vi "ExSubNframeCol_new_recovery_no chart.vi"(8 "error in (no error)":errorcluster, 9 "image handles":u32[](array[numeric]), 10 "Number of Images":u32=1 min=1 step=1, 11 "Handle Cluster 2":T1) -> (0 "error out":errorcluster, 1 "data handles":u32[](array[numeric]), 3 "Handle Cluster":T1, 4 "x > y?":bool, 5 "Frame Rate":dbl=1001.0010010010011, 6 "image #":i32)   [LabVIEW 2015]
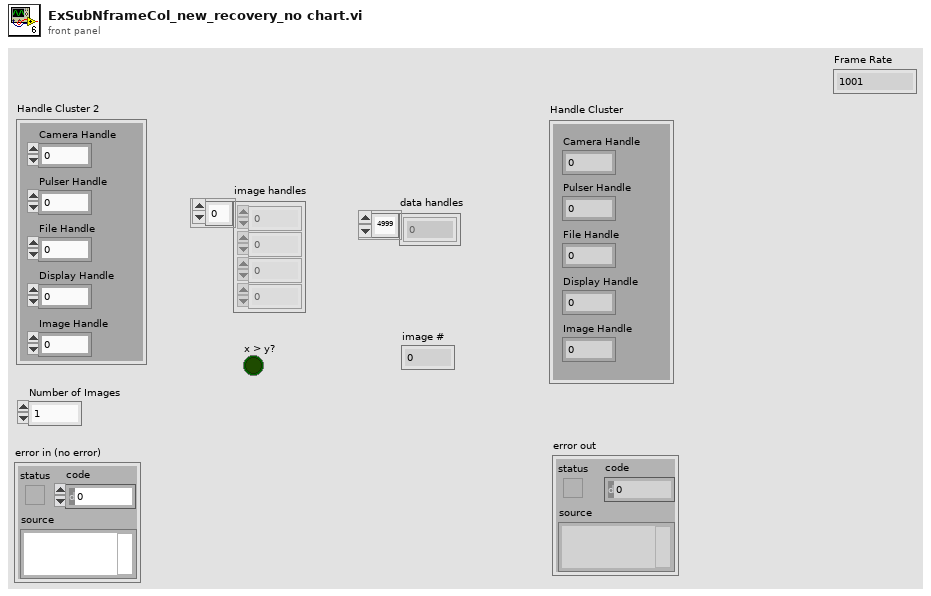
[diagram p1: front panel]
types:
  T1 = cluster{"Camera Handle":u32, "Pulser Handle":u32, "File Handle":u32, "Display Handle":u32, "Image Handle":u32}
  T2 = cluster{"Camera Handle":u32, "Pulser Handle":u32, "File Handle":u32, "Display Handle":u32, "Image/Data Handle":u32}
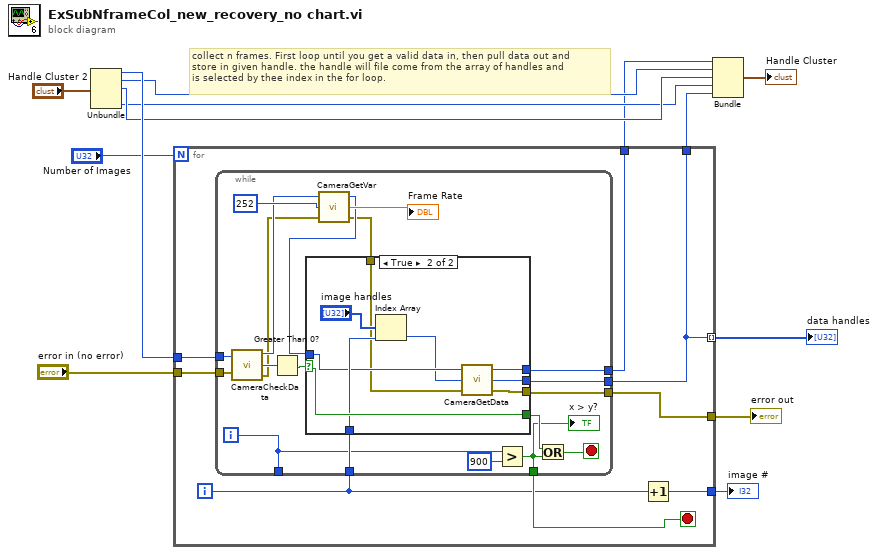
[diagram p0: block diagram]
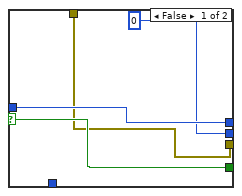
[diagram p2: hidden frame]
diagram:
  # "collect n frames. First loop until you get a valid data in, then pull data out and \nstore in given handle. the handle will file come from the array of handles and\nis selected by thee index in the for loop."
  n1 = Unbundle("Handle Cluster 2") -> ("Camera Handle"=w13:u32, "Pulser Handle"=w10:u32, "File Handle"=w9:u32, "Display Handle"=w8:u32)  [unwired: 1 out]
  n2 = for {
    N: "Number of Images" -> [_]
    tunnel: w13 -> [w21]
    tunnel: "error in (no error)" -> [w20]
    tunnel: [w19] -> w11
    tunnel: [w18] -> w5
    tunnel: [w17] -> w7
    tunnel: [w17] -> w6 mode=indexing
    tunnel: [w14] -> w1
    i -> [w15]
    stop <- w16 stop-if-true
    n3 = while {
      tunnel: w20 -> [w34]
      tunnel: w21 -> [w35]
      tunnel: [w40] -> w19
      tunnel: w15 -> [w39]
      tunnel: [w38] -> w18
      tunnel: [w37] -> w17
      tunnel: [w28] -> _
      tunnel: [w29] -> w16
      i -> [w28]
      stop <- w31 stop-if-true
      n4 = call <userlib>:"CameraCheckData.vi"("Camera Handle"=w35, "error in"=w34) -> ("Camera Handle"=w25:u32, "Number Of Frames Available"=w33:i32, "error out"=w23:errorcluster)
      n5 = Greater Than 0?(x=w33) -> (x > 0?=w36:bool)
      n6 = call <userlib>:"CameraGetVar.vi"("error in"=w23, "Parameter ID"=252, "Camera Handle"=w25) -> ("error out"=w22:errorcluster, "Value"=→"Frame Rate":dbl, "Camera Handle"=w24:u32)
      n7 = case shown="True" w36 {
        selector: w36 -> [w44 w53]
        tunnel: w24 -> [w43 w50]
        tunnel: [w44 w53] -> w32
        tunnel: [w41 w46] -> w40
        tunnel: w39 -> [_ w52]
        tunnel: [w43 w48] -> w38
        tunnel: [0 w47] -> w37
        tunnel: w22 -> [w41 w45]
        frame False {
        }
        frame True {
          n8 = Index Array(array="image handles", index=w52) -> (element=w49:u32)
          n9 = call <userlib>:"CameraGetData.vi"("error in"=w45, "Image/Data Handle"=w49, "Camera Handle"=w50) -> ("error out"=w46:errorcluster, "Image/Data Handle"=w47:u32, "Camera Handle"=w48:u32)
        }
      }
      n10 = Greater?(x=w28, y=900) -> (0:w29:bool)
      "x > y?" <- w29
      n11 = Or(x=w32, y=w29) -> (x .or. y?=w31:bool)
    }
    n12 = Increment(x=w15) -> (x+1=w14:i32)
  }
  "error out" <- w11
  "data handles" <- w6
  "image #" <- w1
  n13 = Bundle("Camera Handle"=w5, "Pulser Handle"=w10, "File Handle"=w9, "Display Handle"=w8, "Image/Data Handle"=w7) -> (→"Handle Cluster":T2)  [unwired: 1 in]
